vi "getAttributeByName.vi"(8 "error in (no error)":errorcluster, 10 "AttributeName":string, 11 "xmlNode in":refnum<class "xmlNode.lvclass">) -> (0 "error out":errorcluster, 2 "attribute string":string, 3 "xmlNode out":refnum<class "xmlNode.lvclass">)   [LabVIEW 2009, in "Tools.lvlib" / "xml.lvlib" / "xmlNode.lvclass"]
uses:
  xmlNode.lvclass
  xmlNode.lvclass/xmlNode.ctl
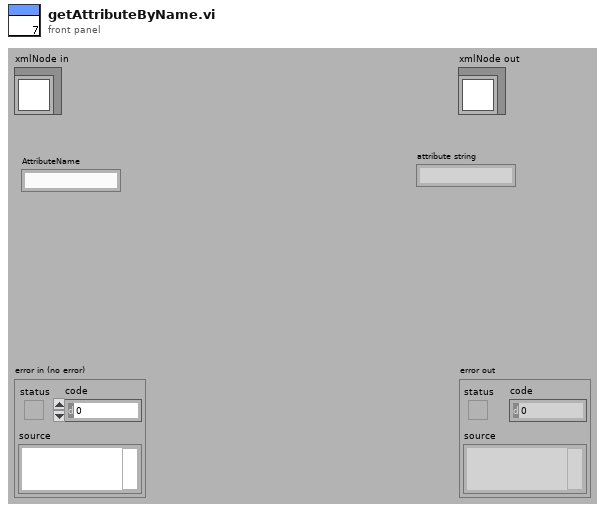
[diagram p1: front panel]
types:
  T1 = cluster{"attribute type":string, "attribute string":string}[]
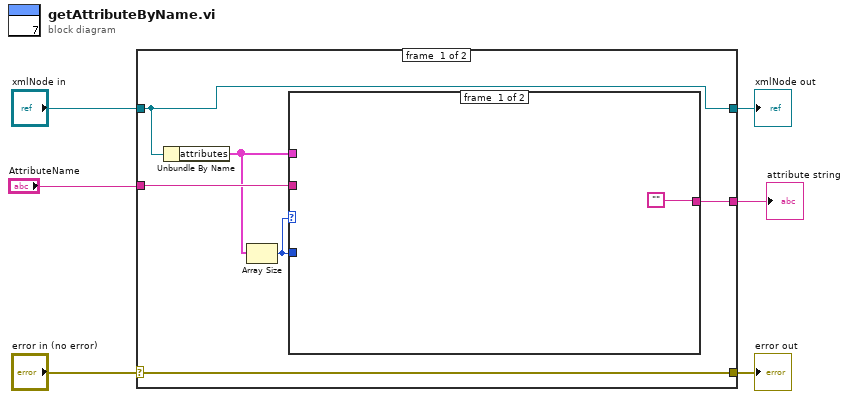
[diagram p0: block diagram]
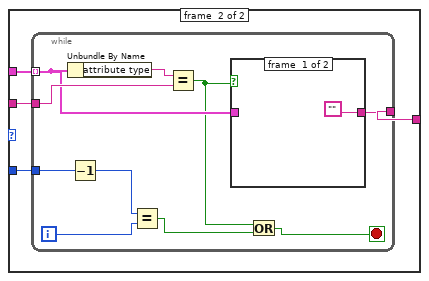
[diagram p2: hidden frame]
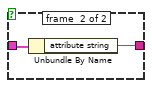
[diagram p3: hidden frame]
diagram:
  n1 = case shown="No Error" "error in (no error)" {
    selector: "error in (no error)" -> [w12 w32]
    tunnel: [w12 w32] -> w5
    tunnel: [w11 w31] -> w3
    tunnel: "xmlNode in" -> [w11 w31]
    tunnel: "AttributeName" -> [w10 _]
    tunnel: [w9 _] -> w1
    frame #0 {
      n2 = Unbundle By Name(w11) -> ("attributes"=w8:T1)
      n3 = Array Size(array=w8) -> (size(s)=w7:i32)
      n4 = case shown="Default" w7 {
        tunnel: w10 -> [_ w17]
        tunnel: ["" w16] -> w9
        tunnel: w8 -> [_ w15]
        tunnel: w7 -> [_ w14]
        frame #0 {
        }
        frame #1 {
          n5 = while {
            tunnel: w15 -> [w25] mode=indexing
            tunnel: w17 -> [w26]
            tunnel: [w24] -> w16
            tunnel: w14 -> [w22]
            i -> [w21]
            stop <- w18 stop-if-true
            n6 = Unbundle By Name(w25) -> ("attribute type"=w27:string)
            n7 = Decrement(x=w22) -> (x-1=w20:i32)
            n8 = Equal?(x=w20, y=w21) -> (x = y?=w19:bool)
            n9 = Equal?(x=w27, y=w26) -> (x = y?=w23:bool)
            n10 = case shown="True" w23 {
              tunnel: w25 -> [_ w30]
              tunnel: ["" w29] -> w24
              frame #0 {
              }
              frame #1 {
                n11 = Unbundle By Name(w30) -> ("attribute string"=w29:string)
              }
            }
            n12 = Or(x=w23, y=w19) -> (x .or. y?=w18:bool)
          }
        }
      }
    }
    frame #1 {
    }
  }
  "error out" <- w5
  "xmlNode out" <- w3
  "attribute string" <- w1
